vi "Read controlTerminals.vi"(8 "error in (no error)":errorcluster, 11 "BlockDiagram in":refnum<class "BlockDiagram.lvclass">) -> (0 "error out":errorcluster, 2 "terminals":refnum<class "Terminal.lvclass">[](array[class]), 3 "BlockDiagram out":refnum<class "BlockDiagram.lvclass">)   [LabVIEW 2023, in "TLC_Scripto.lvlib" / "BlockDiagram.lvclass"]
uses:
  BlockDiagram.lvclass
  BlockDiagram.lvclass/BlockDiagram.ctl
  ControlTerminal/ControlTerminal.lvclass
  C:/projects/TLC_Scripto/Source/Terminal/Terminal.lvclass
  C:/projects/TLC_Scripto/Source/GObject/GObject.lvclass
  C:/projects/TLC_Scripto/Source/Generic/Generic.lvclass
  C:/projects/TLC_Scripto/Source/ControlTerminal/ControlTerminal.lvclass
  Terminal/Terminal.lvclass
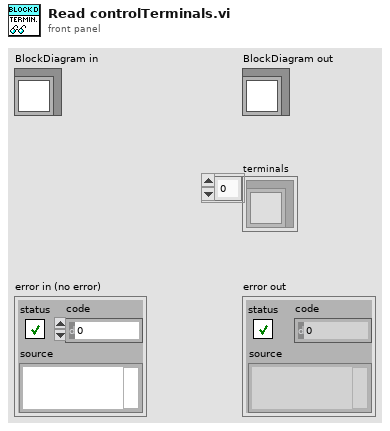
[diagram p1: front panel]
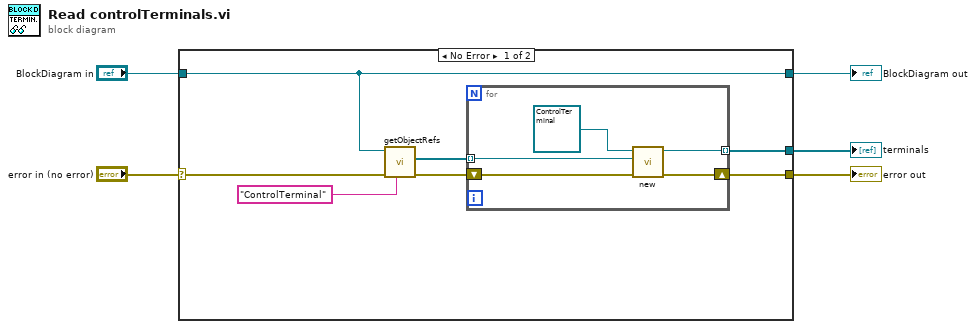
[diagram p0: block diagram]
diagram:
  n1 = case shown="No Error" "error in (no error)" {
    selector: "error in (no error)" -> [w7 w19]
    tunnel: [w9 w19] -> w4
    tunnel: [w10 w18] -> w2
    tunnel: "BlockDiagram in" -> [w10 w18]
    tunnel: [w8 _] -> w1
    frame No Error {
      n2 = call "getObjectRefs.vi"("type(ClassName)"="ControlTerminal", "error in (no error)"=w7, "BlockDiagram in"=w10) -> ("error out"=w11:errorcluster, "refs"=w12:refnum<vi>[])  [unwired: 6 in, 1 out]
      n3 = for {
        tunnel: w12 -> [w17] mode=indexing
        shift-right: [w15] -> w9
        shift-left: w11 -> [w16]
        tunnel: [w14] -> w8 mode=indexing
        n4 = call-dynamic "new.vi"("Error In"=w16, "ref"=w17, "Generic In"=refnum<class "ControlTerminal.lvclass"> refnum ("TLC_Scripto.lvlib:ControlTerminal")) -> ("Error Out"=w15:errorcluster, "Generic Out"=w14:refnum<class "ControlTerminal.lvclass">)  [unwired: 7 in]
      }
    }
    frame Error {
    }
  }
  "error out" <- w4
  "BlockDiagram out" <- w2
  "terminals" <- w1
